vi "Send Read View Settings.vi"(7 "Priority":T1=enum."Normal" caption="Message Priority (Normal)", 8 "error in (no error)":errorcluster, 10 "View Name":string, 11 "Message Enqueuer in":refnum<class "Message Enqueuer.lvclass">) -> (0 "error out":errorcluster, 3 "Message Enqueuer out":refnum<class "Message Enqueuer.lvclass">)   [LabVIEW 2023, in "MVC Actors.lvlib" / "Read View Settings Msg.lvclass"]
doc: "Sends the <b>MVC Actors.lvlib:Read View Settings Msg.lvclass</b> message.\n\nThis message will call <b>Read View Settings.vi</b> on the <b>MVC Actors.lvlib:Controller.lvclass</b> actor.\n\n<b>Read View Settings.vi Description</b>\nAllows the child controller to get the behavior of a View actor specified in the <b>View Name</b> by registering to the user defined event whose reference is accessible by the <b>View Settings Event Ref</b> property that will deliver the following settings\n\n<b>Exclude From Broadcast</b>: message originating form another View will not be broadcasted to the View being cosidered\n<b>Paused</b>: the View will not send events and will not receive them anymore\n<b>Receive only</b>: The View will receive events but not send any"
uses:
  Read View Settings Msg.lvclass
  Read View Settings Msg.lvclass/Read View Settings Msg.ctl
  <vilib>/ActorFramework/Message Enqueuer/Message Enqueuer.lvclass
  C:/Program Files/National Instruments/LabVIEW 2023/vi.lib/ActorFramework/Message/Message.lvclass
  C:/Projects/Shared Libraries/Event Actors/Controller Messages/Read View Settings Msg/Read View Settings Msg.lvclass
  <vilib>/ActorFramework/Message Enqueuer/Message Priority.ctl
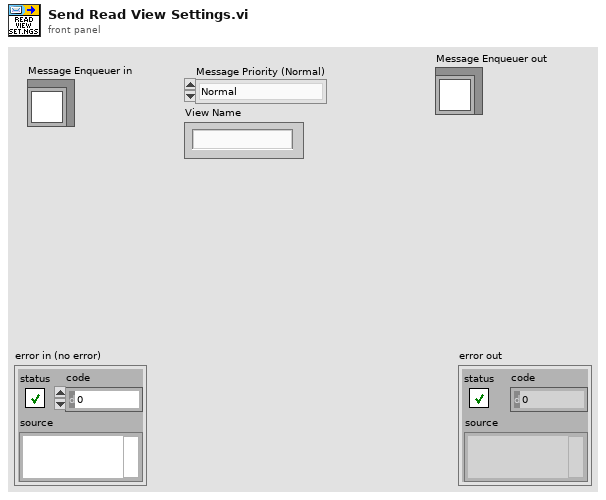
[diagram p1: front panel]
types:
  T1 = typedef "Actor Framework.lvlib/Message Enqueuer.lvclass/Message Priority.ctl" = enum16{"Low", "Normal", "High"}
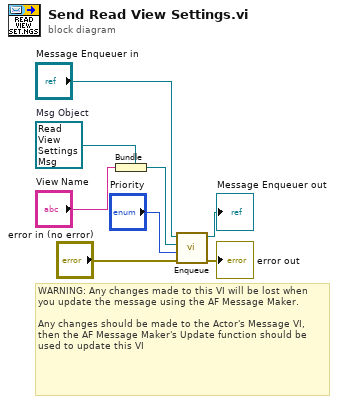
[diagram p0: block diagram]
diagram:
  w7 = refnum<class "Read View Settings Msg.lvclass"> refnum  # Msg Object
  # "WARNING: Any changes made to this VI will be lost when you update the message using the AF Message Maker.\n\nAny changes should be made to the Actor's Message VI, then the AF Message Maker's Update function should be used to update this VI"
  n1 = Bundle(cluster=w7, "View Name") -> (w2:refnum<class "Read View Settings Msg.lvclass">)
  n2 = call <vilib>:"Enqueue.vi"("error in (no error)"="error in (no error)", "Message Priority (Normal)"="Priority", "Message"=w2, "Message Enqueuer in"="Message Enqueuer in") -> ("error out"=→"error out":errorcluster, "Message Enqueuer out"=→"Message Enqueuer out":refnum<class "Message Enqueuer.lvclass">)  [unwired: 6 in]
